vi "主程序-生产消费-1.vi"() -> ()   [LabVIEW 2014]
doc: "该模板用于创建生产者／消费者模式的应用程序，以事件驱动的方式，生成队列中的项。如需通过响应事件实现代码的异步执行，同时不影响用户界面的响应速度，可考虑用该模式替代“用户界面事件处理器”模式。"
uses:
  <vilib>/Instr/_visa.llb/VISA Configure Serial Port (Instr).vi
panel:
  out "读取缓冲区":string
  out "CRC校验位":string
  out "运行速度（256-65535）":i32
  in  "减速（Max=65535）":i32=550 max=65535
  in  "加速（Max=65535）":i32=550 max=65535
  in  "位置控制模式":bool
  in  "行进距离（Max=16777214）":i32=25500 max=16777214
  out "验证":string
  out "abc":string
  in  "执行次数":i32=3
  in  "模式选择":string(combo)="\u0000"
  out "低位":string
  out "高位":string
  in  "速度增减幅度":u16(ring)=1 items=["1"=1, "10"=10, "20"=20, "50"=50, "100"=100, "200"=200, "500"=500, "1000"=1000, "2000"=2000, "5000"=5000, "10000"=10000]
  in  "速度-":bool
  in  "速度+":bool
  in  "运行速度（256-65535）":i32=63500 min=256 max=65535
  in  "停止运行":bool
  in  "负向运行":bool
  in  "正向运行":bool
  in  "停止":bool
  in  "端口开关":bool
  in  "端口选择":refnum<visa-resource-name>
  # "步进电机控制系统"
  # "请关闭端口开关后再停止程序！"
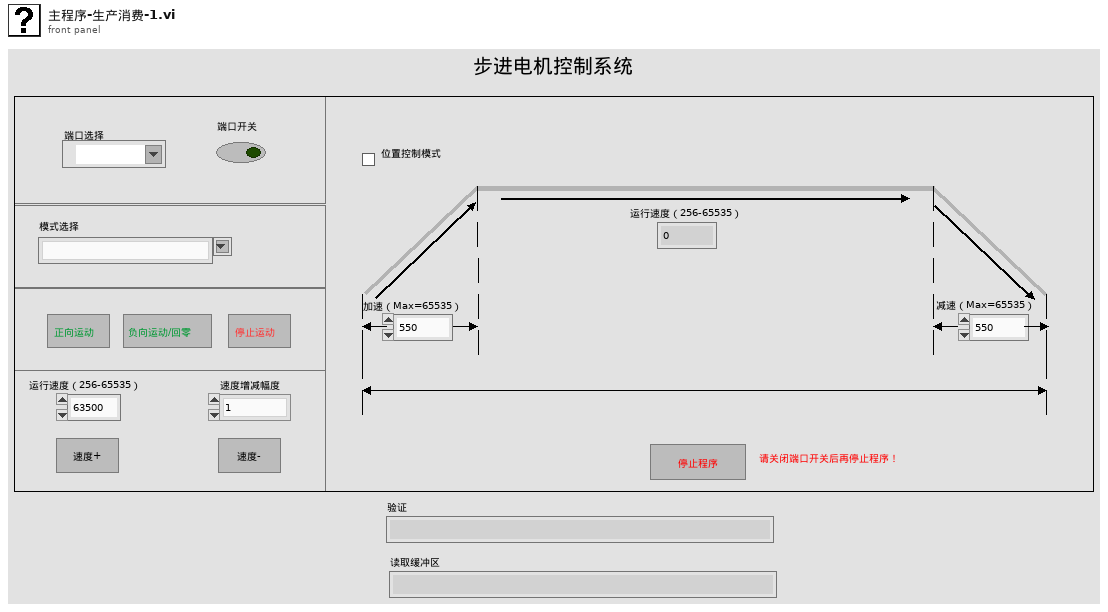
[diagram p1: front panel]
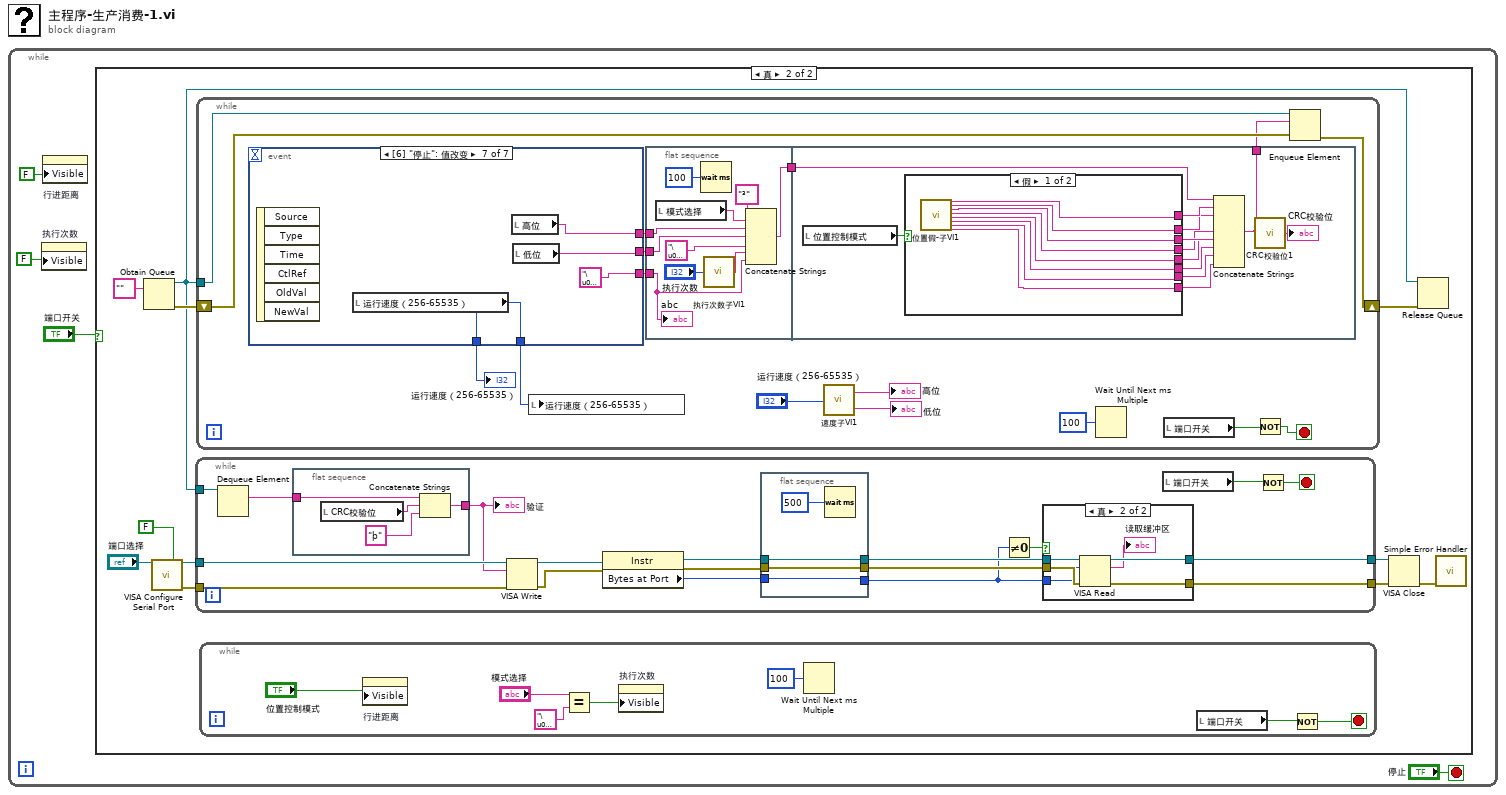
[diagram p0: block diagram]
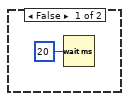
[diagram p2: hidden frame]
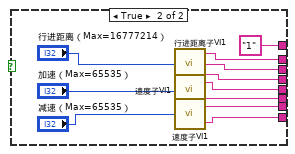
[diagram p4: hidden frame]
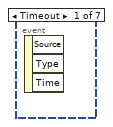
[diagram p5: hidden frame]
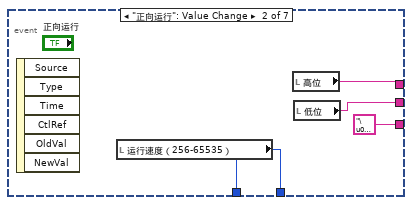
[diagram p6: hidden frame]
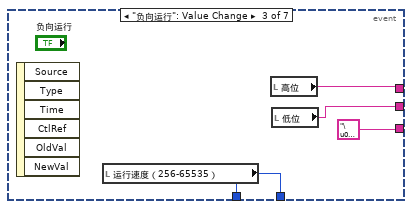
[diagram p7: hidden frame]
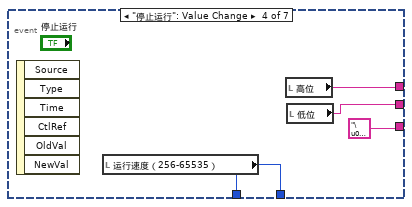
[diagram p8: hidden frame]
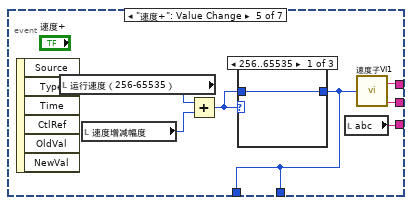
[diagram p9: hidden frame]
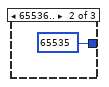
[diagram p10: hidden frame]
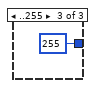
[diagram p11: hidden frame]
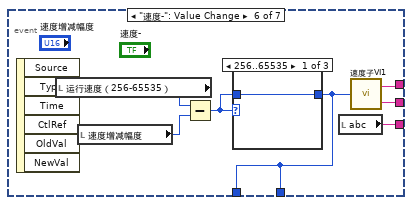
[diagram p12: hidden frame]
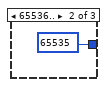
[diagram p13: hidden frame]
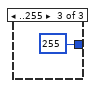
[diagram p14: hidden frame]
diagram:
  n1 = while {
    stop <- "停止" stop-if-true
    n2 = property on="执行次数" class="DigNum (严格)"("Visible"=FALSE) -> ()  [unwired: 2 in, 2 out]
    n3 = property on="行进距离" class="DigNum (严格)"("Visible"=FALSE) -> ()  [unwired: 2 in, 2 out]
    n4 = case shown="真" "端口开关" {
      frame False {
        n5 = Wait (ms)(milliseconds to wait=u32 20 ("等待时间（毫秒）")) -> ()  [unwired: 1 out]
      }
      frame True {
        n6 = Obtain Queue(element data type="") -> (queue out=w7:refnum<queue>, error out=w16:errorcluster)  [unwired: 4 in, 1 out]
        n7 = call-poly "VISA Configure Serial Port"("VISA resource name"="端口选择", "Enable Termination\nChar (T)"=FALSE ("Enable Termination\nChar (T)")) -> ("VISA resource name out"=w13:refnum<visa-resource-name>, "error out"=w12:errorcluster)  [unwired: 12 in]
        n8 = while {
          tunnel: w13 -> [w41]
          tunnel: w12 -> [w40]
          tunnel: [w39] -> w9
          tunnel: [w38] -> w8
          tunnel: w7 -> [w36]
          stop <- w33 stop-if-true
          n9 = Dequeue Element(queue=w36) -> (element=w35:string)  [unwired: 2 in, 3 out]
          n10 = flat-sequence {
            tunnel: [w55] -> w37
            tunnel: w35 -> [w54]
            frame #0 {
              n11 = local read "CRC校验位"() -> (w57:string)
              n12 = Concatenate Strings(w54, w57, "þ" ("字符串")) -> (w55:string)
            }
          }
          n13 = VISA Write(VISA resource name=w41, write buffer=w37, error in (no error)=w40) -> (VISA resource name out=w32:refnum<visa-resource-name>, error out=w31:errorcluster)  [unwired: 1 out]
          n14 = property class="Instr"(reference=w32, error in=w31) -> (reference out=w30:refnum<visa-resource-name>, error out=w29:errorcluster, "Bytes at Port"=w28:u32)
          n15 = flat-sequence {
            tunnel: w30 -> [w53]
            tunnel: [w53] -> w27
            tunnel: w29 -> [w52]
            tunnel: [w52] -> w26
            tunnel: w28 -> [w51]
            tunnel: [w51] -> w24
            frame #0 {
              n16 = Wait (ms)(milliseconds to wait=u32 500 ("等待时间（毫秒）")) -> ()  [unwired: 1 out]
            }
          }
          n17 = Not Equal To 0?(x=w24) -> (x != 0?=w25:bool)
          n18 = case shown="真" w25 {
            tunnel: [w43 w49] -> w39
            tunnel: [w42 w48] -> w38
            tunnel: w27 -> [w43 w46]
            tunnel: w26 -> [w42 w45]
            tunnel: w24 -> [_ w44]
            frame False {
            }
            frame True {
              n19 = VISA Read(VISA resource name=w46, byte count=w44, error in (no error)=w45) -> (VISA resource name out=w49:refnum<visa-resource-name>, read buffer=→"读取缓冲区":string, error out=w48:errorcluster)  [unwired: 1 out]
            }
          }
          n20 = local read "端口开关"() -> (w34:bool)
          n21 = Not(x=w34) -> (.not. x?=w33:bool)
          "验证" <- w37
        }
        n22 = while {
          shift-right: [w68] -> w15
          shift-left: w16 -> [w73]
          tunnel: w7 -> [w72]
          stop <- w58 stop-if-true
          n23 = event shown="[6] \"停止\": 值改变" {
            selector: _ -> [_ _ _ _ _ _ _]
            dyn-events: _ -> [_ _ _ _ _ _ _]
            timeout: _ -> [_ _ _ _ _ _ _]
            tunnel: [_ w118 w122 w126 w130 w140 w148] -> w65
            tunnel: [_ w117 w121 w125 w129 w139 w147] -> w64
            tunnel: [_ "\u0001" "\u0002" "\u0003" w128 w138 "\u0003"] -> w63
            tunnel: [_ w115 w119 w123 w127 w137 w149] -> w67
            tunnel: [_ w115 w119 w123 w127 w137 w149] -> w66
            event Timeout {
              n24 = event-data() -> ()  [unwired: 1 in, 3 out]
            }
            event "正向运行": Value Change {
              n25 = event-data() -> ()  [unwired: 1 in, 6 out]
              n26 = local read "运行速度（256-65535）"() -> (w115:i32)
              n27 = local read "高位"() -> (w118:string)
              n28 = local read "低位"() -> (w117:string)
            }
            event "负向运行": Value Change {
              n29 = event-data() -> ()  [unwired: 1 in, 6 out]
              n30 = local read "运行速度（256-65535）"() -> (w119:i32)
              n31 = local read "高位"() -> (w122:string)
              n32 = local read "低位"() -> (w121:string)
            }
            event "停止运行": Value Change {
              n33 = event-data() -> ()  [unwired: 1 in, 6 out]
              n34 = local read "运行速度（256-65535）"() -> (w123:i32)
              n35 = local read "高位"() -> (w126:string)
              n36 = local read "低位"() -> (w125:string)
            }
            event "速度+": Value Change {
              n37 = event-data() -> ()  [unwired: 1 in, 6 out]
              n38 = local read "运行速度（256-65535）"() -> (w133:i32)
              n39 = local read "速度增减幅度"() -> (w132:u16)
              n40 = Add(x=w133, y=w132) -> (x+y=w131:i32)
              n41 = case shown="256..65535" w131 {
                tunnel: w131 -> [w134 _ _]
                tunnel: [w134 65535 255] -> w127
                frame 256..65535 {
                }
                frame 65536.. {
                }
                frame ..255 {
                }
              }
              n42 = local read "abc"() -> (w128:string)
              n43 = call "速度子VI1.vi"("脉冲数"=w127) -> ("分频基数高位"=w130:string, "分频基数低位"=w129:string)
            }
            event "速度-": Value Change {
              n44 = event-data() -> ()  [unwired: 1 in, 6 out]
              n45 = local read "运行速度（256-65535）"() -> (w143:i32)
              n46 = local read "速度增减幅度"() -> (w142:u16)
              n47 = Subtract(x=w143, y=w142) -> (x-y=w141:i32)
              n48 = case shown="256..65535" w141 {
                tunnel: w141 -> [w144 _ _]
                tunnel: [w144 65535 255] -> w137
                frame 256..65535 {
                }
                frame 65536.. {
                }
                frame ..255 {
                }
              }
              n49 = local read "abc"() -> (w138:string)
              n50 = call "速度子VI1.vi"("脉冲数"=w137) -> ("分频基数高位"=w140:string, "分频基数低位"=w139:string)
            }
            event "停止": Value Change {
              n51 = event-data() -> ()  [unwired: 1 in, 6 out]
              n52 = local read "运行速度（256-65535）"() -> (w149:i32)
              n53 = local read "高位"() -> (w148:string)
              n54 = local read "低位"() -> (w147:string)
            }
          }
          "运行速度（256-65535）" <- w67
          n55 = local write "运行速度（256-65535）"(w66) -> ()
          n56 = flat-sequence {
            tunnel: w65 -> [w82]
            tunnel: w64 -> [w81]
            tunnel: w63 -> [w78]
            tunnel: [w76] -> w61
            tunnel: w61 -> [w86]
            tunnel: [w85] -> w60
            frame #0 {
              n57 = local read "模式选择"() -> (w75:string)
              n58 = Wait (ms)(milliseconds to wait=u32 100 ("毫秒倍数")) -> ()  [unwired: 1 out]
              n59 = call "执行次数子VI1.vi"("执行次数"="执行次数") -> ("HEX显示"=w79:string)
              n60 = Concatenate Strings("³" ("字符串"), w75, w82, w81, "\u0000", w79, w78) -> (w76:string)
              "abc" <- w78
            }
            frame #1 {
              n61 = local read "位置控制模式"() -> (w84:bool)
              n62 = case shown="假" w84 {
                tunnel: [w96 w114] -> w87
                tunnel: [w97 w113] -> w88
                tunnel: [w98 w112] -> w89
                tunnel: [w99 w111] -> w90
                tunnel: [w100 w110] -> w91
                tunnel: [w101 w109] -> w92
                tunnel: [w102 w108] -> w93
                tunnel: [w103 "1"] -> w94
                frame False {
                  n63 = call "位置假-子VI1.vi"() -> ("8"=w103:string, "9"=w102:string, "10"=w101:string, "11"=w100:string, "12"=w99:string, "13"=w98:string, "14"=w97:string, "15"=w96:string)  [unwired: 20 in]
                }
                frame True {
                  n64 = call "行进距离子VI1.vi"("脉冲输入端"="行进距离（Max=16777214）") -> ("行进脉冲总数高位"=w108:string, "行进脉冲总数中位"=w109:string, "行进脉冲总数低位"=w110:string)
                  n65 = call "速度子VI1.vi"("脉冲数"="加速（Max=65535）") -> ("分频基数高位"=w111:string, "分频基数低位"=w112:string)
                  n66 = call "速度子VI1.vi"("脉冲数"="减速（Max=65535）") -> ("分频基数高位"=w113:string, "分频基数低位"=w114:string)
                }
              }
              n67 = Concatenate Strings(w86, w94, w93, w92, w91, w90, w89, w88, w87) -> (w85:string)
              n68 = call "CRC校验位1.vi"("输入端"=w85) -> ("CRC校验位"=→"CRC校验位":string)
            }
          }
          n69 = call "速度子VI1.vi"("脉冲数"="运行速度（256-65535）") -> ("分频基数高位"=→"高位":string, "分频基数低位"=→"低位":string)
          n70 = Wait Until Next ms Multiple(millisecond multiple=u32 100 ("毫秒倍数")) -> ()  [unwired: 1 out]
          n71 = local read "端口开关"() -> (w59:bool)
          n72 = Not(x=w59) -> (.not. x?=w58:bool)
          n73 = Enqueue Element(queue=w72, element=w60, error in (no error)=w73) -> (error out=w68:errorcluster)  [unwired: 1 in, 2 out]
        }
        n74 = while {
          stop <- w18 stop-if-true
          n75 = property on="行进距离" class="DigNum (严格)"("Visible"="位置控制模式") -> ()  [unwired: 2 in, 2 out]
          n76 = Equal?(x="模式选择", y="\u0004") -> (x = y?=w20:bool)
          n77 = property on="执行次数" class="DigNum (严格)"("Visible"=w20) -> ()  [unwired: 2 in, 2 out]
          n78 = Wait Until Next ms Multiple(millisecond multiple=u32 100 ("等待时间（毫秒）")) -> ()  [unwired: 1 out]
          n79 = local read "端口开关"() -> (w19:bool)
          n80 = Not(x=w19) -> (.not. x?=w18:bool)
        }
        n81 = VISA Close(VISA resource name=w9, error in (no error)=w8) -> (error out=w10:errorcluster)
        n82 = Release Queue(queue=w7, error in (no error)=w15) -> ()  [unwired: 1 in, 3 out]
        n83 = call <vilib>:"Simple Error Handler.vi"("error in (no error)"=w10) -> ()  [unwired: 4 in, 5 out]
      }
    }
  }
